vi "exposureTimeMet.vi"(8 "error in (no error)":errorcluster, 11 "Model in":refnum<class "Model.lvclass">) -> (0 "error out":errorcluster, 3 "Model out":refnum<class "Model.lvclass">)   [LabVIEW 2016, in "Model.lvclass"]
uses:
  Model.lvclass
  Typedefs/SubDataSignal.ctl
  ts_sallv_sedspectrometer/DataTypes/command_stopImageCapture.ctl
  Typedefs/SEDSpectrometerTypedefs.lvlib
  ts_sallv_sedspectrometer/SALLV_sedSpectrometer.lvlib
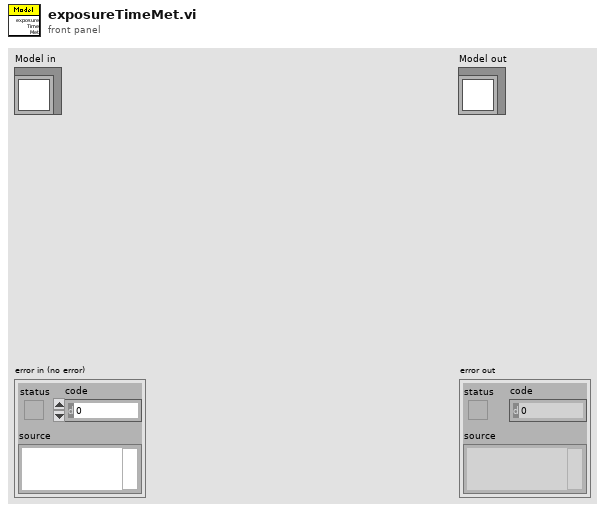
[diagram p1: front panel]
types:
  T1 = typedef "SALLV_sedSpectrometer.lvlib/command_stopImageCapture.ctl" = cluster{"stop":bool}
  T2 = typedef "SEDSpectrometerTypedefs.lvlib/SubDataSignal.ctl" = enum16{"disable", "enable", "exit", "standby", "HeartbeatIn", "start", "captureSpectImage", "setSpectTempSetpoint", "stopImageCapture"}
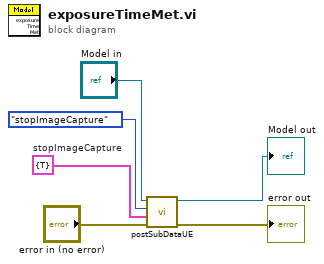
[diagram p0: block diagram]
diagram:
  w4 = T1 {"stop"=TRUE}  # stopImageCapture
  n1 = call "postSubDataUE.vi"("error in (no error)"="error in (no error)", "value"=w4, "subDataSV"=SubDataSignal."stopImageCapture", "Model in"="Model in") -> ("error out"=→"error out":errorcluster, "Model out"=→"Model out":refnum<class "Model.lvclass">)  [unwired: 6 in]
